vi "Run.vi"(8 "error in (no error)":errorcluster, 11 "SPARC4_GUI in":refnum<class "SPARC4_GUI.lvclass">) -> (0 "error out":errorcluster, 3 "SPARC4_GUI out":refnum<class "SPARC4_GUI.lvclass">)   [LabVIEW 2018, in "SPARC4_GUI.lvclass"]
uses:
  SPARC4_GUI.lvclass
  SPARC4_GUI.lvclass/SPARC4_GUI.ctl
  Channel GUI/Channel GUI.lvclass
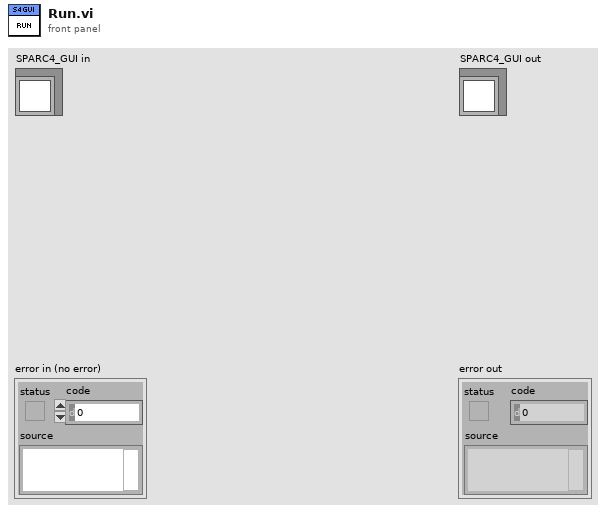
[diagram p1: front panel]
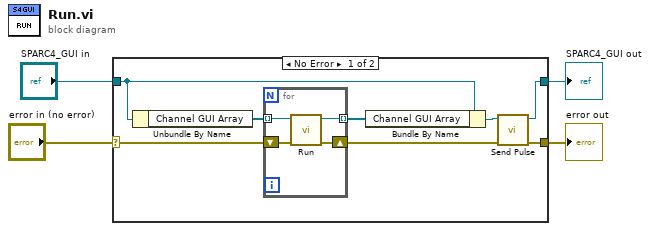
[diagram p0: block diagram]
diagram:
  n1 = case shown="No Error" "error in (no error)" {
    selector: "error in (no error)" -> [w11 w18]
    tunnel: [w6 w18] -> w3
    tunnel: [w7 w17] -> w1
    tunnel: "SPARC4_GUI in" -> [w10 w17]
    frame No Error {
      n2 = Unbundle By Name(w10) -> ("Channel GUI Array"=w12:refnum<class "Channel GUI.lvclass">[])
      n3 = for {
        tunnel: w12 -> [w16] mode=indexing
        tunnel: [w14] -> w9 mode=indexing
        shift-right: [w13] -> w5
        shift-left: w11 -> [w15]
        n4 = call "Run.vi"("error in (no error)"=w15, "Channel GUI in"=w16) -> ("error out"=w13:errorcluster, "Channel GUI out"=w14:refnum<class "Channel GUI.lvclass">)  [unwired: 8 in]
      }
      n5 = Bundle By Name(cluster=w10, "Channel GUI Array"=w9) -> (w8:refnum<class "SPARC4_GUI.lvclass">)
      n6 = call "Send Pulse.vi"("error in (no error)"=w5, "SPARC4_GUI in"=w8) -> ("error out"=w6:errorcluster, "SPARC4_GUI out"=w7:refnum<class "SPARC4_GUI.lvclass">)  [unwired: 8 in]
    }
    frame Error {
    }
  }
  "error out" <- w3
  "SPARC4_GUI out" <- w1
